vi "Teleop.vi"(10 "Match Info":T2={"Autonomous Elapsed Seconds"=0.0, "TeleOp Elapsed Seconds"=0.0, "Disabled Elapsed Seconds"=0.0, "Visited Autonomous"=FALSE, "Visited TeleOp"=FALSE, "Visited Disabled"=FALSE, "Autonomous Settings"={"Autonomous Style"=enum."Independent", "VI Refnum"=refnum}}, 11 "Call Context":T3) -> ()   [LabVIEW 2018]
doc: "This VI is called for each enabled TeleOp packet received from the DS. It is typically used to read from joysticks and other inputs and update I/O or setpoints for timed control loops. It should complete and return within 20 milliseconds or risk missing DS packets."
uses:
  <vilib>/Rock Robotics/WPI/DriverStation/WPI_DriverStationDerivedRobotMode.ctl
  <vilib>/Rock Robotics/WPI/DriverStation/WPI_DriverStationMatch Info.ctl
  <vilib>/Rock Robotics/WPI/Solenoid/WPI_SolenoidValue.ctl
  <vilib>/Rock Robotics/WPI/Utilities/WPI_GetSetVariantRefNum.vi
  <vilib>/Rock Robotics/Network Tables/NT Write Boolean Array.vi
  <vilib>/Rock Robotics/Network Tables/NT Write Numeric Array.vi
  <vilib>/Rock Robotics/Network Tables/NT Write Boolean.vi
  <vilib>/Rock Robotics/WPI/ThirdParty/Phoenix-LabVIEW/Motor Controller/Get/CTRE_Phoenix_MotorController_GetSelectedSensorData.vi
  <vilib>/Rock Robotics/Network Tables/NT Write Number.vi
  <vilib>/Rock Robotics/WPI/Ultrasonic/WPI_SonarSRF04DigitalRefNum Registry Get.vi
  <vilib>/Rock Robotics/WPI/Ultrasonic/WPI_SonarSRF04DigitalGetRange.vi
  <vilib>/Rock Robotics/WPI/RobotDrive/WPI_RobotDriveMecanumDrive_Cartesian.vi
  <vilib>/Rock Robotics/WPI/Solenoid/Deprecated/WPI_SolenoidSetBool.vi
  <vilib>/Rock Robotics/WPI/RobotDrive/WPI_RobotDriveArcadeDrive_Standard(NoSaturation).vi
  <vilib>/Rock Robotics/WPI/Solenoid/WPI_SolenoidSetEnum.vi
panel:
  out "YRPHfH 2":T1
  out "YRPHfH":T1
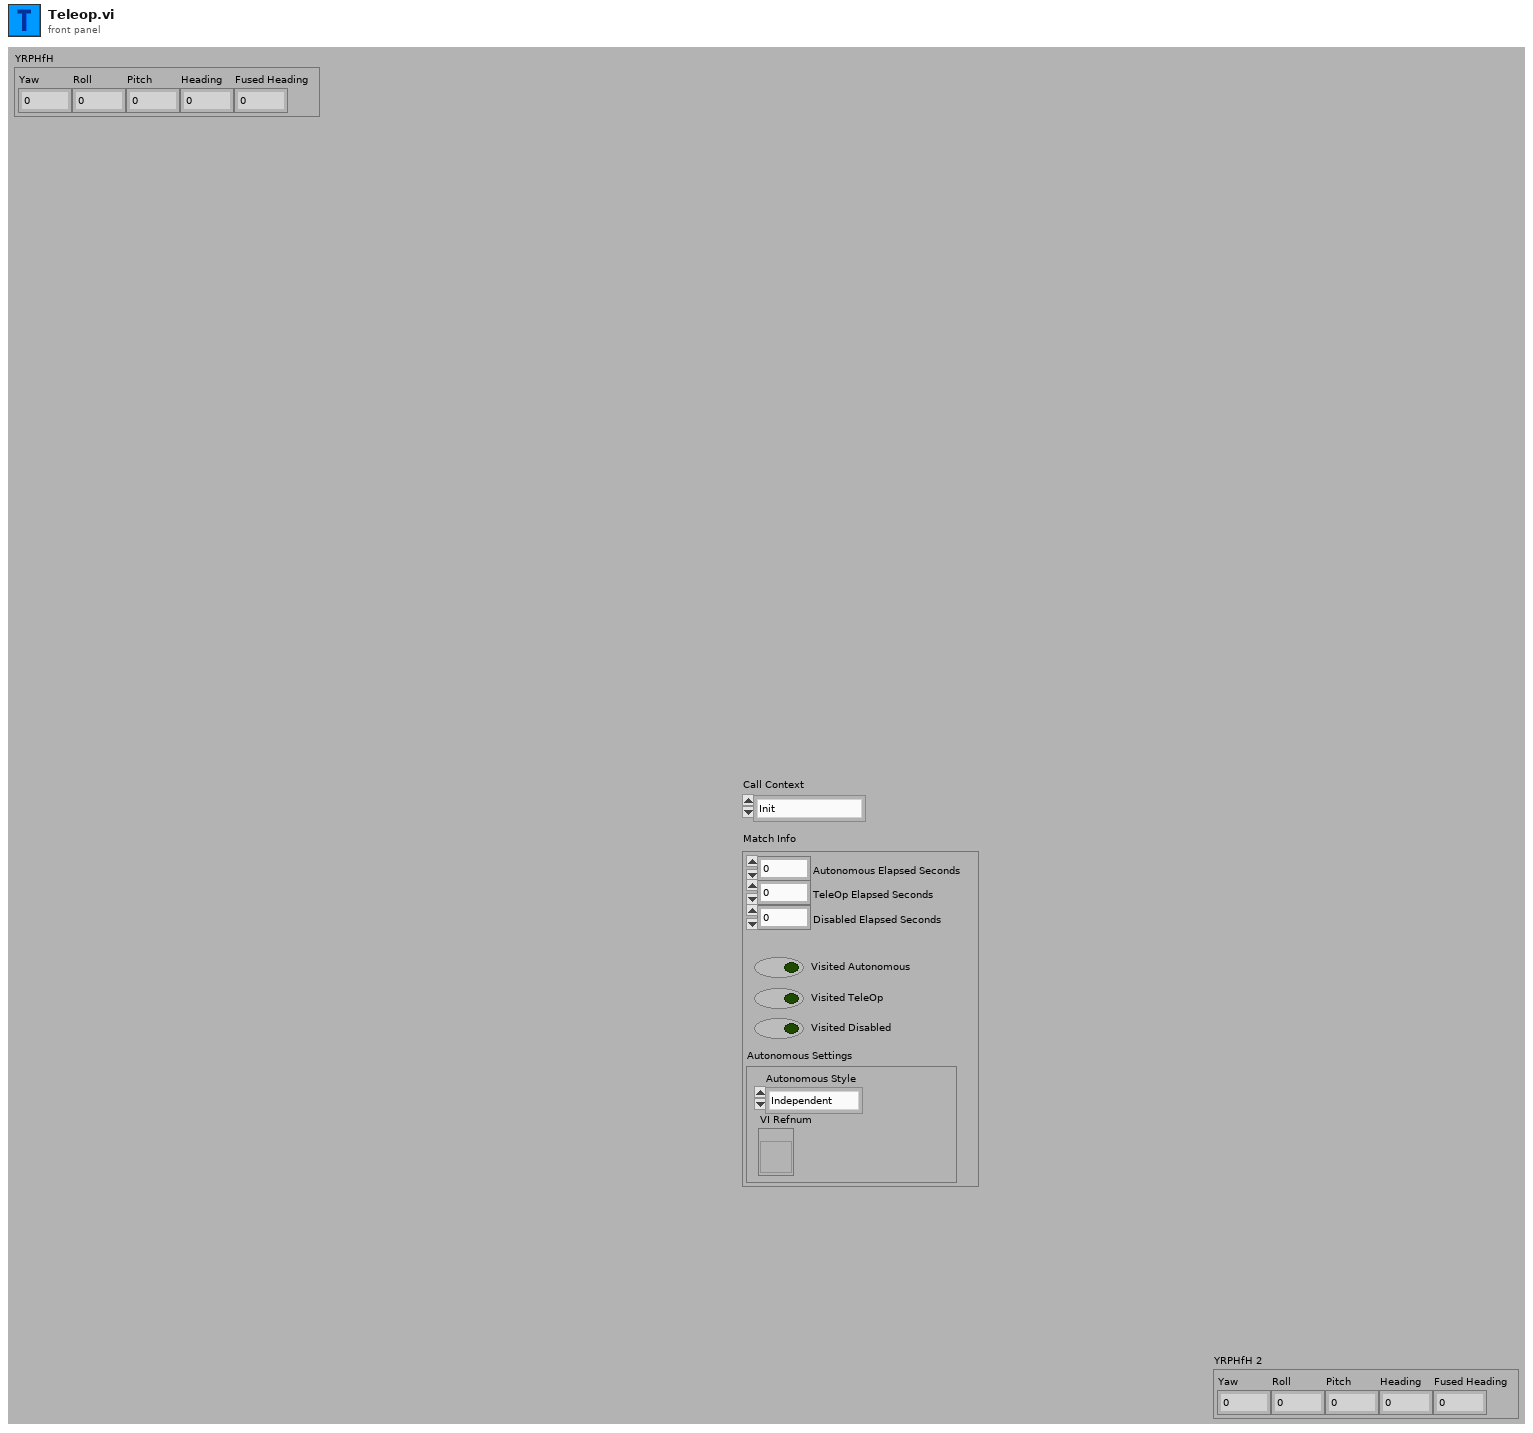
[diagram p1: front panel]
types:
  T1 = cluster{"Yaw":dbl, "Roll":dbl, "Pitch":dbl, "Heading":dbl, "Fused Heading":dbl}
  T2 = typedef "WPI_DriverStationMatch Info.ctl" = cluster{"Autonomous Elapsed Seconds":dbl, "TeleOp Elapsed Seconds":dbl, "Disabled Elapsed Seconds":dbl, "Visited Autonomous":bool, "Visited TeleOp":bool, "Visited Disabled":bool, "Autonomous Settings":cluster{"Autonomous Style":enum16{"Iterative", "Independent"}, "VI Refnum":refnum<vi>}}
  T3 = typedef "WPI_DriverStationDerivedRobotMode.ctl" = enum16{"Init", "Execute", "Stop"}
  T4 = typedef "WPI_MotorControlDeviceRef.ctl" = cluster{"DeviceStatus":errorcluster, "Type":T5, "PWM":cluster{"PWM Channel":T6, "DeadBand":T7}, "CAN":cluster{"Device Number":u8, "SetOutput VI Ref":variant, "GetOutput VI Ref":variant, "Enable VI Ref":variant, "Disable VI Ref":variant, "Data":variant}, "Invert":bool, "DIO PWM":cluster{"PWM \"Enable\" Channel":T6, "DIOChannel":T8, "PWM Rate":dbl}}
  T5 = typedef "WPI_MotorControlType.ctl" = enum16{"PWM", "CAN", "DIO PWM"}
  T6 = typedef "FPGA_DIOPWMChannel.ctl" = enum8{"PWM 0", "PWM 1", "PWM 2", "PWM 3", "PWM 4", "PWM 5", "PWM 6", "PWM 7", "PWM 8", "PWM 9", "PWM MXP 0", "PWM MXP 1", "PWM MXP 2", "PWM MXP 3", "PWM MXP 4", "PWM MXP 5", "PWM MXP 6", "PWM MXP 7", "PWM MXP 8", "PWM MXP 9", "Invalid"}
  T7 = typedef "WPI_PWMDeadband.ctl" = cluster{"Name":string, "maxPositivePwm":i32, "minPositivePwm":i32, "centerPwm":i32, "maxNegativePwm":i32, "minNegativePwm":i32, "angularRange":u16}
  T8 = typedef "FPGA_DIOChannel.ctl" = enum8{"DIO 0", "DIO 1", "DIO 2", "DIO 3", "DIO 4", "DIO 5", "DIO 6", "DIO 7", "DIO 8", "DIO 9", "DIO MXP 0", "DIO MXP 1", "DIO MXP 2", "DIO MXP 3", "DIO MXP 4", "DIO MXP 5", "DIO MXP 6", "DIO MXP 7", "DIO MXP 8", "DIO MXP 9", "DIO MXP 10", "DIO MXP 11", "DIO MXP 12", "DIO MXP 13", "DIO MXP 14", "DIO MXP 15", "SPI Port CS1", "SPI Port CS2", "SPI Port CS3", "SPI Port MISO", "SPI Port MOSI", "Invalid"}
  T9 = typedef "WPI_JoystickDevRef.ctl" = cluster{"Device":T10}
  T10 = typedef "WPI_JoystickDeviceEnum.ctl" = enum16{"USB 0", "USB 1", "USB 2", "USB 3", "USB 4", "USB 5"}
  T11 = typedef "WPI_UltrasonicDeviceRef.ctl" = cluster{"DevStatus":errorcluster, "Ping Channel":T8, "Echo Channel":T8, "CntIndex":T12}
  T12 = typedef "FPGA_CounterCtrSystemIndex.ctl" = enum8{"Ctr 0", "Ctr 1", "Ctr 2", "Ctr 3", "Ctr 4", "Ctr 5", "Ctr 6", "Ctr 7", "Invalid"}
  T13 = typedef "WPI_CompressorDevRef.ctl" = cluster{"DevStatus":errorcluster, "Pneumatics Control Module":u8}
  T14 = typedef "WPI_SolenoidValue.ctl" = enum16{"Off", "On", "Forward", "Reverse"}
  T15 = typedef "WPI_SolenoidDevRef.ctl" = cluster{"DevStatus":errorcluster, "Pneumatics Control Module":u8, "Forward Solenoid Channel":T16, "Reverse Solenoid Channel":T16}
  T16 = typedef "WPI_SolenoidChannel.ctl" = enum8{"Solenoid 0", "Solenoid 1", "Solenoid 2", "Solenoid 3", "Solenoid 4", "Solenoid 5", "Solenoid 6", "Solenoid 7", "Invalid"}
  T17 = typedef "Command Status Info.ctl" = cluster{"Name":string, "Status":T18, "notifier out":T19}
  T18 = typedef "Completion Status.ctl" = enum16{"Successful", "Aborted", "Incomplete"}
  T19 = typedef "Completion Notifier.ctl" = refnum<notifier>
  T20 = typedef "WPI_SwitchDevRef.ctl" = cluster{"DevStatus":errorcluster, "DIO Channel":T8, "CntIndex":T12, "Normally Closed":bool}
  T21 = typedef "WPI_RobotDriveDevRef.ctl" = cluster{"DevStatus":errorcluster, "Motors[]":T4[], "Square Inputs":bool, "Max Output":dbl}
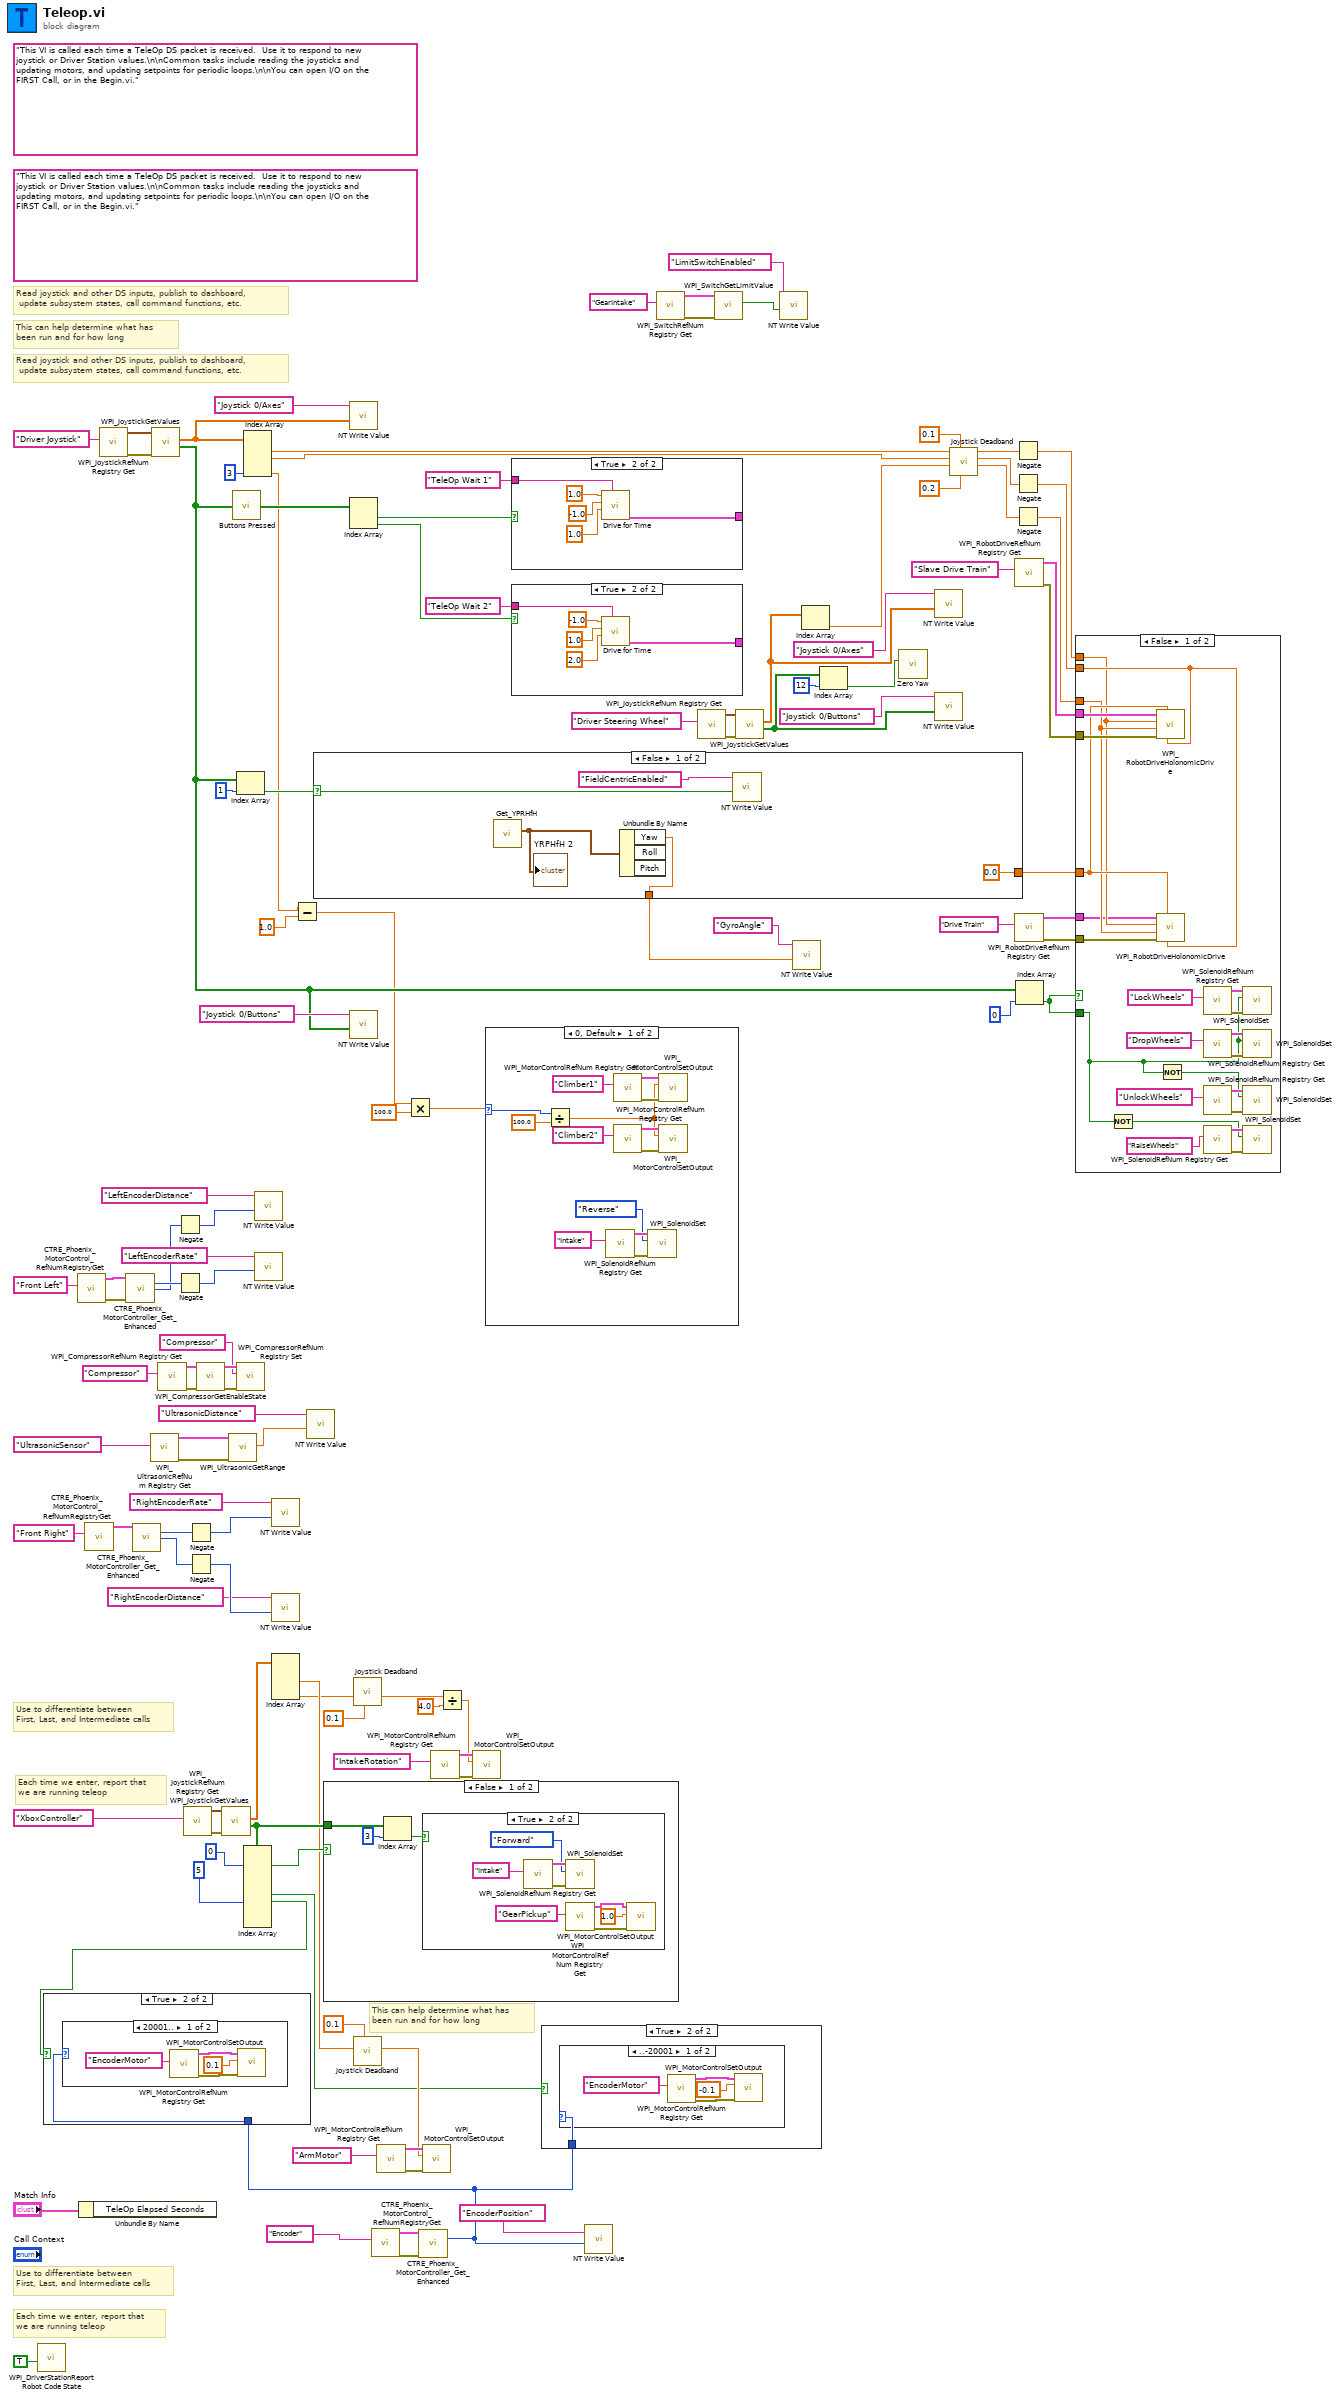
[diagram p0: block diagram]
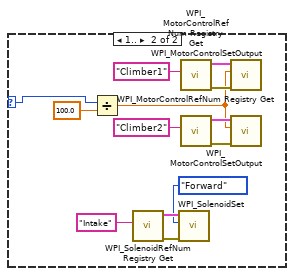
[diagram p2: hidden frame]
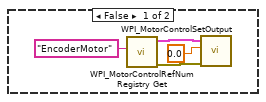
[diagram p3: hidden frame]
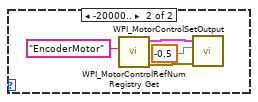
[diagram p4: hidden frame]
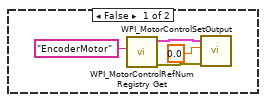
[diagram p5: hidden frame]
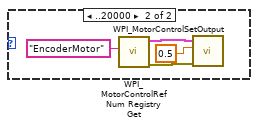
[diagram p6: hidden frame]
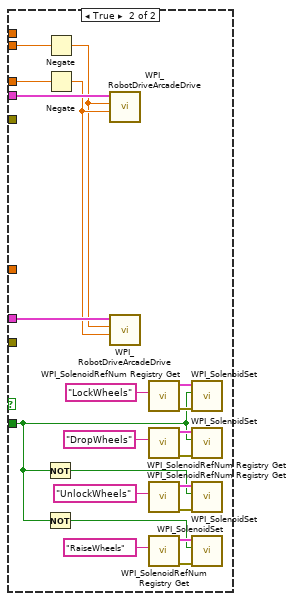
[diagram p7: hidden frame]
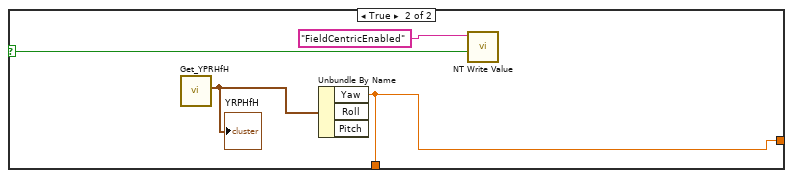
[diagram p8: hidden frame]
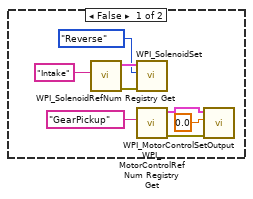
[diagram p9: hidden frame]
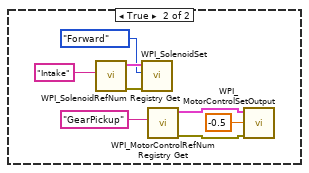
[diagram p10: hidden frame]
diagram:
  (unwired) "This VI is called each time a TeleOp DS packet is received.  Use it to respond to new joystick or Driver Station values.\n\nCommon tasks include reading the joysticks and updating motors, and updating setpoints for periodic loops.\n\nYou can open I/O on the FIRST Call, or in the Begin.vi."
  (unwired) "This VI is called each time a TeleOp DS packet is received.  Use it to respond to new joystick or Driver Station values.\n\nCommon tasks include reading the joysticks and updating motors, and updating setpoints for periodic loops.\n\nYou can open I/O on the FIRST Call, or in the Begin.vi."
  # "Read joystick and other DS inputs, publish to dashboard,\n update subsystem states, call command functions, etc."
  # "Each time we enter, report that\nwe are running teleop"
  # "Use to differentiate between\nFirst, Last, and Intermediate calls"
  # "This can help determine what has\nbeen run and for how long"
  # "Read joystick and other DS inputs, publish to dashboard,\n update subsystem states, call command functions, etc."
  # "Each time we enter, report that\nwe are running teleop"
  # "Use to differentiate between\nFirst, Last, and Intermediate calls"
  # "This can help determine what has\nbeen run and for how long"
  n1 = call <vilib>:"WPI_DriverStationReport Robot Code State.vi"("TeleOp"=TRUE ("Autonomous")) -> ()  [unwired: 10 in, 1 out]
  n2 = call <vilib>:"CTRE_Phoenix_MotorControl_RefNumRegistryGet.vi"("refnum name"="Front Left") -> ("error out"=w82:errorcluster, "PhoenixMotorControlDevRef"=w83:T4)  [unwired: 9 in]
  n3 = Unbundle By Name("Match Info") -> ()  [unwired: 1 out]
  n4 = call <vilib>:"CTRE_Phoenix_MotorControl_RefNumRegistryGet.vi"("refnum name"="Front Right") -> ("PhoenixMotorControlDevRef"=w79:T4)  [unwired: 9 in, 1 out]
  n5 = call <vilib>:"WPI_JoystickRefNum Registry Get.vi"("refnum name"="Driver Joystick") -> ("error out"=w100:errorcluster, "JoystickDevRef"=w112:T9)  [unwired: 1 in, 8 out]
  n6 = call-poly <vilib>:"CTRE_Phoenix_MotorController_Get_Enhanced.vi"("PhoenixMotorControlDevRef"=w83, "error in"=w82) -> ("Position (Raw Sensor Units)"=w81:i32, "Velocity (Raw Sensor Units per 100 ms)"=w71:i32)  [unwired: 10 in, 2 out]
  n7 = call-poly <vilib>:"CTRE_Phoenix_MotorController_Get_Enhanced.vi"("PhoenixMotorControlDevRef"=w79) -> ("Position (Raw Sensor Units)"=w75:i32, "Velocity (Raw Sensor Units per 100 ms)"=w74:i32)  [unwired: 11 in, 2 out]
  n8 = call-poly <vilib>:"WPI_UltrasonicRefNum Registry Get.vi"("refnum name"="UltrasonicSensor") -> ("error out"=w67:errorcluster, "SonarSRF04DevRef"=w68:T11)  [unwired: 9 in]
  n9 = call <vilib>:"WPI_JoystickGetValues.vi"("error in (no error)"=w100, "JoystickDevRef"=w112) -> ("Buttons"=w37:bool[], "Axes"=w105:dbl[])  [unwired: 5 in, 3 out]
  n10 = call <vilib>:"WPI_CompressorRefNum Registry Get.vi"("refnum name"="Compressor") -> ("error out"=w8:errorcluster, "CompressorDevRef"=w11:T13)  [unwired: 9 in]
  n11 = Negate(x=w71) -> (-x=w72:i32)
  n12 = Negate(x=w81) -> (-x=w80:i32)
  n13 = call <vilib>:"WPI_JoystickRefNum Registry Get.vi"("refnum name"="XboxController") -> ("error out"=w62:errorcluster, "JoystickDevRef"=w61:T9)  [unwired: 9 in]
  n14 = Negate(x=w75) -> (-x=w77:i32)
  n15 = Negate(x=w74) -> (-x=w76:i32)
  n16 = call <vilib>:"WPI_CompressorGetEnableState.vi"("error in (no error)"=w8, "CompressorDevRef"=w11) -> ("error out"=w9:errorcluster, "CompressorDevRef"=w10:T13)  [unwired: 6 in, 2 out]
  n17 = call <vilib>:"WPI_JoystickGetValues.vi"("error in (no error)"=w62, "JoystickDevRef"=w61) -> ("Buttons"=w55:bool[], "Axes"=w57:dbl[])  [unwired: 5 in, 3 out]
  n18 = call-poly <vilib>:"WPI_UltrasonicGetRange.vi"("error in (no error)"=w67, "SonarSRF04DevRef"=w68) -> ("Distance"=w66:dbl)  [unwired: 7 in, 2 out]
  n19 = call "Buttons Pressed.vi"("Button Values"=w37) -> ("Button Presses"=w109:bool[])
  n20 = Index Array(array=w37, index=1) -> (element=w43:bool)
  n21 = call <vilib>:"WPI_CompressorRefNum Registry Set.vi"("error in (no error)"=w9, "refnum name"="Compressor", "CompressorDevRef"=w10) -> ()  [unwired: 7 in, 2 out]
  n22 = Index Array(array=w105, index #4=3 ("index")) -> (element #1=w95:dbl, element #2=w94:dbl, element #4=w27:dbl)  [unwired: 3 in, 1 out]
  n23 = Index Array(array=w55, index #1=0, index #6=5 ("index")) -> (element #1=w56:bool, element #5=w18:bool, element #6=w19:bool)  [unwired: 7 in, 6 out]
  n24 = call-poly <vilib>:"NT Write Value.vi"("Numeric"=w72, "Name"="LeftEncoderDistance") -> ()  [unwired: 9 in, 1 out]
  n25 = call-poly <vilib>:"NT Write Value.vi"("Numeric"=w80, "Name"="LeftEncoderRate") -> ()  [unwired: 9 in, 1 out]
  n26 = call-poly <vilib>:"NT Write Value.vi"("Numeric"=w77, "Name"="RightEncoderRate") -> ()  [unwired: 9 in, 1 out]
  n27 = call-poly <vilib>:"NT Write Value.vi"("Numeric"=w76, "Name"="RightEncoderDistance") -> ()  [unwired: 9 in, 1 out]
  n28 = Index Array(array=w57) -> (element #2=w54:dbl, element #4=w48:dbl)  [unwired: 4 in, 2 out]
  n29 = Subtract(x=w27, y=1.0) -> (x-y=w17:dbl)
  n30 = call-poly <vilib>:"NT Write Value.vi"("Numeric"=w66, "Name"="UltrasonicDistance") -> ()  [unwired: 9 in, 1 out]
  n31 = case shown="False" w43 {
    selector: w43 -> [w119 w122]
    tunnel: [0.0 w121] -> w14
    tunnel: [w116 w121] -> w12
    frame False {
      n32 = call <vilib>:"Get_YPRHfH.vi"() -> ("YRPHfH"=w117:T1)  [unwired: 11 in]
      "YRPHfH 2" <- w117
      n33 = Unbundle By Name(w117) -> ("Yaw"=w116:dbl)  [unwired: 2 out]
      n34 = call-poly <vilib>:"NT Write Value.vi"("Boolean"=w119, "Name"="FieldCentricEnabled") -> ()  [unwired: 9 in, 1 out]
    }
    frame True {
      n35 = call <vilib>:"Get_YPRHfH.vi"() -> ("YRPHfH"=w124:T1)  [unwired: 11 in]
      "YRPHfH" <- w124
      n36 = Unbundle By Name(w124) -> ("Yaw"=w121:dbl)  [unwired: 2 out]
      n37 = call-poly <vilib>:"NT Write Value.vi"("Boolean"=w122, "Name"="FieldCentricEnabled") -> ()  [unwired: 9 in, 1 out]
    }
  }
  n38 = case shown="False" w56 {
    tunnel: w55 -> [w126 _]
    frame False {
      n39 = Index Array(array=w126, index=3) -> (element=w125:bool)
      n40 = case shown="True" w125 {
        frame False {
          n41 = call <vilib>:"WPI_SolenoidRefNum Registry Get.vi"("refnum name"="Intake") -> ("error out"=w131:errorcluster, "SolenoidDevRef"=w130:T15)  [unwired: 9 in]
          n42 = call-poly <vilib>:"WPI_SolenoidSet.vi"("error in (no error)"=w131, "Value"=WPI_SolenoidValue."Reverse", "SolenoidDevRef"=w130) -> ()  [unwired: 7 in, 2 out]
          n43 = call <vilib>:"WPI_MotorControlRefNum Registry Get.vi"("refnum name"="GearPickup") -> ("error out"=w135:errorcluster, "MotorControlDevRef"=w134:T4)  [unwired: 9 in]
          n44 = call <vilib>:"WPI_MotorControlSetOutput.vi"("error in (no error)"=w135, "Output"=0.0, "MotorControlDevRef"=w134) -> ()  [unwired: 6 in, 3 out]
        }
        frame True {
          n45 = call <vilib>:"WPI_SolenoidRefNum Registry Get.vi"("refnum name"="Intake") -> ("error out"=w139:errorcluster, "SolenoidDevRef"=w140:T15)  [unwired: 9 in]
          n46 = call-poly <vilib>:"WPI_SolenoidSet.vi"("error in (no error)"=w139, "Value"=WPI_SolenoidValue."Forward", "SolenoidDevRef"=w140) -> ()  [unwired: 7 in, 2 out]
          n47 = call <vilib>:"WPI_MotorControlRefNum Registry Get.vi"("refnum name"="GearPickup") -> ("error out"=w142:errorcluster, "MotorControlDevRef"=w143:T4)  [unwired: 9 in]
          n48 = call <vilib>:"WPI_MotorControlSetOutput.vi"("error in (no error)"=w142, "Output"=1.0, "MotorControlDevRef"=w143) -> ()  [unwired: 6 in, 3 out]
        }
      }
    }
    frame True {
      n49 = call <vilib>:"WPI_SolenoidRefNum Registry Get.vi"("refnum name"="Intake") -> ("error out"=w147:errorcluster, "SolenoidDevRef"=w145:T15)  [unwired: 9 in]
      n50 = call-poly <vilib>:"WPI_SolenoidSet.vi"("error in (no error)"=w147, "Value"=WPI_SolenoidValue."Forward", "SolenoidDevRef"=w145) -> ()  [unwired: 7 in, 2 out]
      n51 = call <vilib>:"WPI_MotorControlRefNum Registry Get.vi"("refnum name"="GearPickup") -> ("error out"=w148:errorcluster, "MotorControlDevRef"=w149:T4)  [unwired: 9 in]
      n52 = call <vilib>:"WPI_MotorControlSetOutput.vi"("error in (no error)"=w148, "Output"=-0.5, "MotorControlDevRef"=w149) -> ()  [unwired: 6 in, 3 out]
    }
  }
  n53 = call-poly <vilib>:"NT Write Value.vi"("Numeric Array"=w105, "Name"="Joystick 0/Axes") -> ()  [unwired: 9 in, 1 out]
  n54 = Index Array(array=w109) -> (element #1=w108:bool, element #2=w107:bool)  [unwired: 2 in]
  n55 = call-poly <vilib>:"NT Write Value.vi"("Boolean Array"=w37, "Name"="Joystick 0/Buttons") -> ()  [unwired: 9 in, 1 out]
  n56 = call "Joystick Deadband.vi"("Z Deadband"=0.1, "Z"=w48) -> ("Z Out"=w45:dbl)  [unwired: 7 in, 2 out]
  n57 = call "Joystick Deadband.vi"("X Y Deadband"=0.1, "Y"=w54) -> ("Y Out"=w52:dbl)  [unwired: 7 in, 2 out]
  n58 = call <vilib>:"CTRE_Phoenix_MotorControl_RefNumRegistryGet.vi"("refnum name"="Encoder") -> ("error out"=w23:errorcluster, "PhoenixMotorControlDevRef"=w24:T4)  [unwired: 9 in]
  n59 = call <vilib>:"WPI_MotorControlRefNum Registry Get.vi"("refnum name"="ArmMotor") -> ("error out"=w59:errorcluster, "MotorControlDevRef"=w58:T4)  [unwired: 9 in]
  n60 = Multiply(x=w17, y=100.0) -> (x*y=w15:dbl)
  n61 = call-poly <vilib>:"CTRE_Phoenix_MotorController_Get_Enhanced.vi"("PhoenixMotorControlDevRef"=w24, "error in"=w23) -> ("Position (Raw Sensor Units)"=w20:i32)  [unwired: 10 in, 3 out]
  n62 = case shown="True" w19 {
    tunnel: w20 -> [_ w156]
    frame False {
      n63 = call <vilib>:"WPI_MotorControlRefNum Registry Get.vi"("refnum name"="EncoderMotor") -> ("error out"=w155:errorcluster, "MotorControlDevRef"=w154:T4)  [unwired: 9 in]
      n64 = call <vilib>:"WPI_MotorControlSetOutput.vi"("error in (no error)"=w155, "Output"=0.0, "MotorControlDevRef"=w154) -> ()  [unwired: 6 in, 3 out]
    }
    frame True {
      n65 = case shown="20001.." w156 {
        frame 20001.. {
          n66 = call <vilib>:"WPI_MotorControlRefNum Registry Get.vi"("refnum name"="EncoderMotor") -> ("error out"=w159:errorcluster, "MotorControlDevRef"=w160:T4)  [unwired: 9 in]
          n67 = call <vilib>:"WPI_MotorControlSetOutput.vi"("error in (no error)"=w159, "Output"=0.1, "MotorControlDevRef"=w160) -> ()  [unwired: 6 in, 3 out]
        }
        frame ..20000 {
          n68 = call <vilib>:"WPI_MotorControlRefNum Registry Get.vi"("refnum name"="EncoderMotor") -> ("error out"=w163:errorcluster, "MotorControlDevRef"=w161:T4)  [unwired: 9 in]
          n69 = call <vilib>:"WPI_MotorControlSetOutput.vi"("error in (no error)"=w163, "Output"=0.5, "MotorControlDevRef"=w161) -> ()  [unwired: 6 in, 3 out]
        }
      }
    }
  }
  n70 = call <vilib>:"WPI_MotorControlSetOutput.vi"("error in (no error)"=w59, "Output"=w52, "MotorControlDevRef"=w58) -> ()  [unwired: 6 in, 3 out]
  n71 = call <vilib>:"WPI_MotorControlRefNum Registry Get.vi"("refnum name"="IntakeRotation") -> ("error out"=w51:errorcluster, "MotorControlDevRef"=w50:T4)  [unwired: 9 in]
  n72 = Divide(x=w45, y=4.0) -> (x/y=w44:dbl)
  n73 = call <vilib>:"WPI_MotorControlSetOutput.vi"("error in (no error)"=w51, "Output"=w44, "MotorControlDevRef"=w50) -> ()  [unwired: 6 in, 3 out]
  n74 = case shown="0, Default" w15 {
    selector: w15 -> [w166 w179]
    frame 0, Default {
      n75 = Divide(x=w166, y=100.0) -> (x/y=w165:dbl)
      n76 = call <vilib>:"WPI_SolenoidRefNum Registry Get.vi"("refnum name"="Intake") -> ("error out"=w177:errorcluster, "SolenoidDevRef"=w176:T15)  [unwired: 9 in]
      n77 = call <vilib>:"WPI_MotorControlRefNum Registry Get.vi"("refnum name"="Climber1") -> ("error out"=w170:errorcluster, "MotorControlDevRef"=w171:T4)  [unwired: 9 in]
      n78 = call <vilib>:"WPI_MotorControlRefNum Registry Get.vi"("refnum name"="Climber2") -> ("error out"=w172:errorcluster, "MotorControlDevRef"=w173:T4)  [unwired: 9 in]
      n79 = call-poly <vilib>:"WPI_SolenoidSet.vi"("error in (no error)"=w177, "Value"=WPI_SolenoidValue."Reverse", "SolenoidDevRef"=w176) -> ()  [unwired: 7 in, 2 out]
      n80 = call <vilib>:"WPI_MotorControlSetOutput.vi"("error in (no error)"=w170, "Output"=w165, "MotorControlDevRef"=w171) -> ()  [unwired: 6 in, 3 out]
      n81 = call <vilib>:"WPI_MotorControlSetOutput.vi"("error in (no error)"=w172, "Output"=w165, "MotorControlDevRef"=w173) -> ()  [unwired: 6 in, 3 out]
    }
    frame 1.. {
      n82 = Divide(x=w179, y=100.0) -> (x/y=w178:dbl)
      n83 = call <vilib>:"WPI_SolenoidRefNum Registry Get.vi"("refnum name"="Intake") -> ("error out"=w183:errorcluster, "SolenoidDevRef"=w184:T15)  [unwired: 9 in]
      n84 = call-poly <vilib>:"WPI_SolenoidSet.vi"("error in (no error)"=w183, "Value"=WPI_SolenoidValue."Forward", "SolenoidDevRef"=w184) -> ()  [unwired: 7 in, 2 out]
      n85 = call <vilib>:"WPI_MotorControlRefNum Registry Get.vi"("refnum name"="Climber1") -> ("error out"=w189:errorcluster, "MotorControlDevRef"=w188:T4)  [unwired: 9 in]
      n86 = call <vilib>:"WPI_MotorControlRefNum Registry Get.vi"("refnum name"="Climber2") -> ("error out"=w186:errorcluster, "MotorControlDevRef"=w185:T4)  [unwired: 9 in]
      n87 = call <vilib>:"WPI_MotorControlSetOutput.vi"("error in (no error)"=w189, "Output"=w178, "MotorControlDevRef"=w188) -> ()  [unwired: 6 in, 3 out]
      n88 = call <vilib>:"WPI_MotorControlSetOutput.vi"("error in (no error)"=w186, "Output"=w178, "MotorControlDevRef"=w185) -> ()  [unwired: 6 in, 3 out]
    }
  }
  n89 = case shown="True" w108 {
    tunnel: [_ w194] -> _
    tunnel: "TeleOp Wait 1" ("Description") -> [_ w193]
    frame False {
    }
    frame True {
      n90 = call "Drive for Time.vi"("Description"=w193, "Seconds"=1.0, "Right Speed"=-1.0, "Left Speed"=1.0) -> ("Command Info Out"=w194:T17)  [unwired: 6 in, 1 out]
    }
  }
  n91 = case shown="True" w107 {
    tunnel: [_ w198] -> _
    tunnel: "TeleOp Wait 2" ("Description") -> [_ w197]
    frame False {
    }
    frame True {
      n92 = call "Drive for Time.vi"("Description"=w197, "Seconds"=2.0, "Right Speed"=1.0, "Left Speed"=-1.0) -> ("Command Info Out"=w198:T17)  [unwired: 6 in, 1 out]
    }
  }
  n93 = case shown="True" w18 {
    tunnel: w20 -> [_ w205]
    frame False {
      n94 = call <vilib>:"WPI_MotorControlRefNum Registry Get.vi"("refnum name"="EncoderMotor") -> ("error out"=w204:errorcluster, "MotorControlDevRef"=w203:T4)  [unwired: 9 in]
      n95 = call <vilib>:"WPI_MotorControlSetOutput.vi"("error in (no error)"=w204, "Output"=0.0, "MotorControlDevRef"=w203) -> ()  [unwired: 6 in, 3 out]
    }
    frame True {
      n96 = case shown="..-20001" w205 {
        frame ..-20001 {
          n97 = call <vilib>:"WPI_MotorControlRefNum Registry Get.vi"("refnum name"="EncoderMotor") -> ("error out"=w208:errorcluster, "MotorControlDevRef"=w209:T4)  [unwired: 9 in]
          n98 = call <vilib>:"WPI_MotorControlSetOutput.vi"("error in (no error)"=w208, "Output"=-0.1, "MotorControlDevRef"=w209) -> ()  [unwired: 6 in, 3 out]
        }
        frame -20000.. {
          n99 = call <vilib>:"WPI_MotorControlRefNum Registry Get.vi"("refnum name"="EncoderMotor") -> ("error out"=w212:errorcluster, "MotorControlDevRef"=w210:T4)  [unwired: 9 in]
          n100 = call <vilib>:"WPI_MotorControlSetOutput.vi"("error in (no error)"=w212, "Output"=-0.5, "MotorControlDevRef"=w210) -> ()  [unwired: 6 in, 3 out]
        }
      }
    }
  }
  n101 = call-poly <vilib>:"NT Write Value.vi"("Numeric"=w20, "Name"="EncoderPosition") -> ()  [unwired: 9 in, 1 out]
  n102 = call <vilib>:"WPI_SwitchRefNum Registry Get.vi"("refnum name"="GearIntake") -> ("error out"=w4:errorcluster, "SwitchDevRef"=w5:T20)  [unwired: 9 in]
  n103 = call <vilib>:"WPI_JoystickRefNum Registry Get.vi"("refnum name"="Driver Steering Wheel") -> ("error out"=w102:errorcluster, "JoystickDevRef"=w101:T9)  [unwired: 9 in]
  n104 = call <vilib>:"WPI_SwitchGetLimitValue.vi"("error in (no error)"=w4, "SwitchDevRef"=w5) -> ("Switch Pressed"=w2:bool)  [unwired: 7 in, 2 out]
  n105 = call <vilib>:"WPI_JoystickGetValues.vi"("error in (no error)"=w102, "JoystickDevRef"=w101) -> ("Buttons"=w89:bool[], "Axes"=w97:dbl[])  [unwired: 5 in, 3 out]
  n106 = call-poly <vilib>:"NT Write Value.vi"("Boolean"=w2, "Name"="LimitSwitchEnabled") -> ()  [unwired: 9 in, 1 out]
  n107 = call-poly <vilib>:"NT Write Value.vi"("Numeric"=w12, "Name"="GyroAngle") -> ()  [unwired: 9 in, 1 out]
  n108 = Index Array(array=w97) -> (element=w93:dbl)  [unwired: 1 in]
  n109 = Index Array(array=w89, index=12) -> (element=w88:bool)
  n110 = call <vilib>:"Zero Yaw.vi"("Zero"=w88) -> ()  [unwired: 11 in]
  n111 = call-poly <vilib>:"NT Write Value.vi"("Numeric Array"=w97, "Name"="Joystick 0/Axes") -> ()  [unwired: 9 in, 1 out]
  n112 = call-poly <vilib>:"NT Write Value.vi"("Boolean Array"=w89, "Name"="Joystick 0/Buttons") -> ()  [unwired: 9 in, 1 out]
  n113 = call "Joystick Deadband.vi"("Z Deadband"=0.2, "X Y Deadband"=0.1, "Z"=w93, "Y"=w94, "X"=w95) -> ("Z Out"=w40:dbl, "Y Out"=w41:dbl, "X Out"=w39:dbl)  [unwired: 4 in]
  n114 = Negate(x=w39) -> (-x=w32:dbl)
  n115 = Negate(x=w41) -> (-x=w35:dbl)
  n116 = Negate(x=w40) -> (-x=w33:dbl)
  n117 = call <vilib>:"WPI_RobotDriveRefNum Registry Get.vi"("refnum name"="Slave Drive Train") -> ("error out"=w34:errorcluster, "RobotDriveDevRef"=w31:T21)  [unwired: 9 in]
  n118 = call <vilib>:"WPI_RobotDriveRefNum Registry Get.vi"("refnum name"="Drive Train") -> ("error out"=w30:errorcluster, "RobotDriveDevRef"=w29:T21)  [unwired: 9 in]
  n119 = Index Array(array=w37, index=0) -> (element=w36:bool)
  n120 = case shown="False" w36 {
    tunnel: w36 -> [w214 w237]
    tunnel: w35 -> [w234 w246]
    tunnel: w14 -> [w233 _]
    tunnel: w34 -> [w236 _]
    tunnel: w33 -> [w231 w247]
    tunnel: w32 -> [w230 _]
    tunnel: w31 -> [w235 w250]
    tunnel: w30 -> [w232 _]
    tunnel: w29 -> [w229 w251]
    frame False {
      n121 = Not(x=w214) -> (.not. x?=w221:bool)
      n122 = call-poly <vilib>:"WPI_RobotDriveHolonomicDrive.vi"("Rotation"=w234, "Gyro Angle"=w233, "error in (no error)"=w236, "Y"=w231, "X"=w230, "RobotDriveDevRef"=w235) -> ()  [unwired: 3 in, 3 out]
      n123 = call-poly <vilib>:"WPI_RobotDriveHolonomicDrive.vi"("Rotation"=w234, "Gyro Angle"=w233, "error in (no error)"=w232, "Y"=w231, "X"=w230, "RobotDriveDevRef"=w229) -> ()  [unwired: 3 in, 3 out]
      n124 = Not(x=w214) -> (.not. x?=w225:bool)
      n125 = call <vilib>:"WPI_SolenoidRefNum Registry Get.vi"("refnum name"="LockWheels") -> ("error out"=w217:errorcluster, "SolenoidDevRef"=w216:T15)  [unwired: 9 in]
      n126 = call <vilib>:"WPI_SolenoidRefNum Registry Get.vi"("refnum name"="DropWheels") -> ("error out"=w220:errorcluster, "SolenoidDevRef"=w219:T15)  [unwired: 9 in]
      n127 = call <vilib>:"WPI_SolenoidRefNum Registry Get.vi"("refnum name"="UnlockWheels") -> ("error out"=w228:errorcluster, "SolenoidDevRef"=w227:T15)  [unwired: 9 in]
      n128 = call <vilib>:"WPI_SolenoidRefNum Registry Get.vi"("refnum name"="RaiseWheels") -> ("error out"=w224:errorcluster, "SolenoidDevRef"=w223:T15)  [unwired: 9 in]
      n129 = call-poly <vilib>:"WPI_SolenoidSet.vi"("error in (no error)"=w217, "Value"=w214, "SolenoidDevRef"=w216) -> ()  [unwired: 7 in, 2 out]
      n130 = call-poly <vilib>:"WPI_SolenoidSet.vi"("error in (no error)"=w220, "Value"=w214, "SolenoidDevRef"=w219) -> ()  [unwired: 7 in, 2 out]
      n131 = call-poly <vilib>:"WPI_SolenoidSet.vi"("error in (no error)"=w228, "Value"=w225, "SolenoidDevRef"=w227) -> ()  [unwired: 7 in, 2 out]
      n132 = call-poly <vilib>:"WPI_SolenoidSet.vi"("error in (no error)"=w224, "Value"=w221, "SolenoidDevRef"=w223) -> ()  [unwired: 7 in, 2 out]
    }
    frame True {
      n133 = Not(x=w237) -> (.not. x?=w242:bool)
      n134 = Not(x=w237) -> (.not. x?=w238:bool)
      n135 = Negate(x=w246) -> (-x=w248:dbl)
      n136 = Negate(x=w247) -> (-x=w249:dbl)
      n137 = call-poly <vilib>:"WPI_RobotDriveArcadeDrive.vi"("Y axis value"=w249, "X axis value"=w248, "RobotDriveDevRef"=w250) -> ()  [unwired: 6 in, 3 out]
      n138 = call-poly <vilib>:"WPI_RobotDriveArcadeDrive.vi"("Y axis value"=w249, "X axis value"=w248, "RobotDriveDevRef"=w251) -> ()  [unwired: 6 in, 3 out]
      n139 = call <vilib>:"WPI_SolenoidRefNum Registry Get.vi"("refnum name"="LockWheels") -> ("error out"=w254:errorcluster, "SolenoidDevRef"=w253:T15)  [unwired: 9 in]
      n140 = call <vilib>:"WPI_SolenoidRefNum Registry Get.vi"("refnum name"="DropWheels") -> ("error out"=w257:errorcluster, "SolenoidDevRef"=w256:T15)  [unwired: 9 in]
      n141 = call <vilib>:"WPI_SolenoidRefNum Registry Get.vi"("refnum name"="UnlockWheels") -> ("error out"=w245:errorcluster, "SolenoidDevRef"=w244:T15)  [unwired: 9 in]
      n142 = call <vilib>:"WPI_SolenoidRefNum Registry Get.vi"("refnum name"="RaiseWheels") -> ("error out"=w241:errorcluster, "SolenoidDevRef"=w240:T15)  [unwired: 9 in]
      n143 = call-poly <vilib>:"WPI_SolenoidSet.vi"("error in (no error)"=w254, "Value"=w237, "SolenoidDevRef"=w253) -> ()  [unwired: 7 in, 2 out]
      n144 = call-poly <vilib>:"WPI_SolenoidSet.vi"("error in (no error)"=w257, "Value"=w237, "SolenoidDevRef"=w256) -> ()  [unwired: 7 in, 2 out]
      n145 = call-poly <vilib>:"WPI_SolenoidSet.vi"("error in (no error)"=w245, "Value"=w242, "SolenoidDevRef"=w244) -> ()  [unwired: 7 in, 2 out]
      n146 = call-poly <vilib>:"WPI_SolenoidSet.vi"("error in (no error)"=w241, "Value"=w238, "SolenoidDevRef"=w240) -> ()  [unwired: 7 in, 2 out]
    }
  }
